vi "Talon Encoder Rotate New.vi"(4 "Right Rotations":dbl, 5 "Right Speed":dbl, 6 "Left Rotations":dbl, 7 "Left Speed":dbl, 9 "RightEncoderMotorRef":T1={"DeviceStatus"={"status"=FALSE, "code"=0, "source"=""}, "Type"=enum."PWM", "PWM"={"PWM Channel"=enum."Invalid", "DeadBand"={"Name"="", "maxPositivePwm"=0, "minPositivePwm"=0, "centerPwm"=0, "maxNegativePwm"=0, "minNegativePwm"=0, "angularRange"=0}}, "CAN"={"Device Number"=0, "Control Mode"=enum."Percent VBus", "Semaphore"=refnum, "Max Vout"=12.0, "TalonSRX Control Mode"=enum."Percent VBus"}, "Invert"=FALSE}, 10 "LeftEncoderMotorRef":T1={"DeviceStatus"={"status"=FALSE, "code"=0, "source"=""}, "Type"=enum."PWM", "PWM"={"PWM Channel"=enum."Invalid", "DeadBand"={"Name"="", "maxPositivePwm"=0, "minPositivePwm"=0, "centerPwm"=0, "maxNegativePwm"=0, "minNegativePwm"=0, "angularRange"=0}}, "CAN"={"Device Number"=0, "Control Mode"=enum."Percent VBus", "Semaphore"=refnum, "Max Vout"=12.0, "TalonSRX Control Mode"=enum."Percent VBus"}, "Invert"=FALSE}, 11 "RobotDriveDevRef":T8={"DevStatus"={"status"=FALSE, "code"=0, "source"=""}, "Motors[]"=[], "Square Inputs"=FALSE, "Max Output"=1.0}) -> (1 "RightEncoderMotorRef":T1={"DeviceStatus"={"status"=FALSE, "code"=0, "source"=""}, "Type"=enum."PWM", "PWM"={"PWM Channel"=enum."Invalid", "DeadBand"={"Name"="", "maxPositivePwm"=0, "minPositivePwm"=0, "centerPwm"=0, "maxNegativePwm"=0, "minNegativePwm"=0, "angularRange"=0}}, "CAN"={"Device Number"=0, "Control Mode"=enum."Percent VBus", "Semaphore"=refnum, "Max Vout"=12.0, "TalonSRX Control Mode"=enum."Percent VBus"}, "Invert"=FALSE}, 2 "LeftEncoderMotorRef":T1={"DeviceStatus"={"status"=FALSE, "code"=0, "source"=""}, "Type"=enum."PWM", "PWM"={"PWM Channel"=enum."Invalid", "DeadBand"={"Name"="", "maxPositivePwm"=0, "minPositivePwm"=0, "centerPwm"=0, "maxNegativePwm"=0, "minNegativePwm"=0, "angularRange"=0}}, "CAN"={"Device Number"=0, "Control Mode"=enum."Percent VBus", "Semaphore"=refnum, "Max Vout"=12.0, "TalonSRX Control Mode"=enum."Percent VBus"}, "Invert"=FALSE}, 3 "RobotDriveDevRef":T8={"DevStatus"={"status"=FALSE, "code"=0, "source"=""}, "Motors[]"=[], "Square Inputs"=FALSE, "Max Output"=1.0})   [LabVIEW 2015]
uses:
  <vilib>/Rock Robotics/WPI/MotorControl/WPI_MotorControlDeviceRef.ctl
  <vilib>/Rock Robotics/WPI/MotorControl/WPI_MotorControlType.ctl
  <vilib>/Rock Robotics/SystemInterfaces/DIO/FPGA_DIOPWMChannel.ctl
  <vilib>/Rock Robotics/WPI/PWM/WPI_PWMDeadband.ctl
  <vilib>/Rock Robotics/WPI/CAN/Jaguar/SubVIs/WPI_CANJaguar_ControlMode.ctl
  <vilib>/Rock Robotics/WPI/CAN/TalonSRX/WPI_CANTalonSRX_APIControlMode.ctl
  <vilib>/Rock Robotics/WPI/RobotDrive/WPI_RobotDriveDevRef.ctl
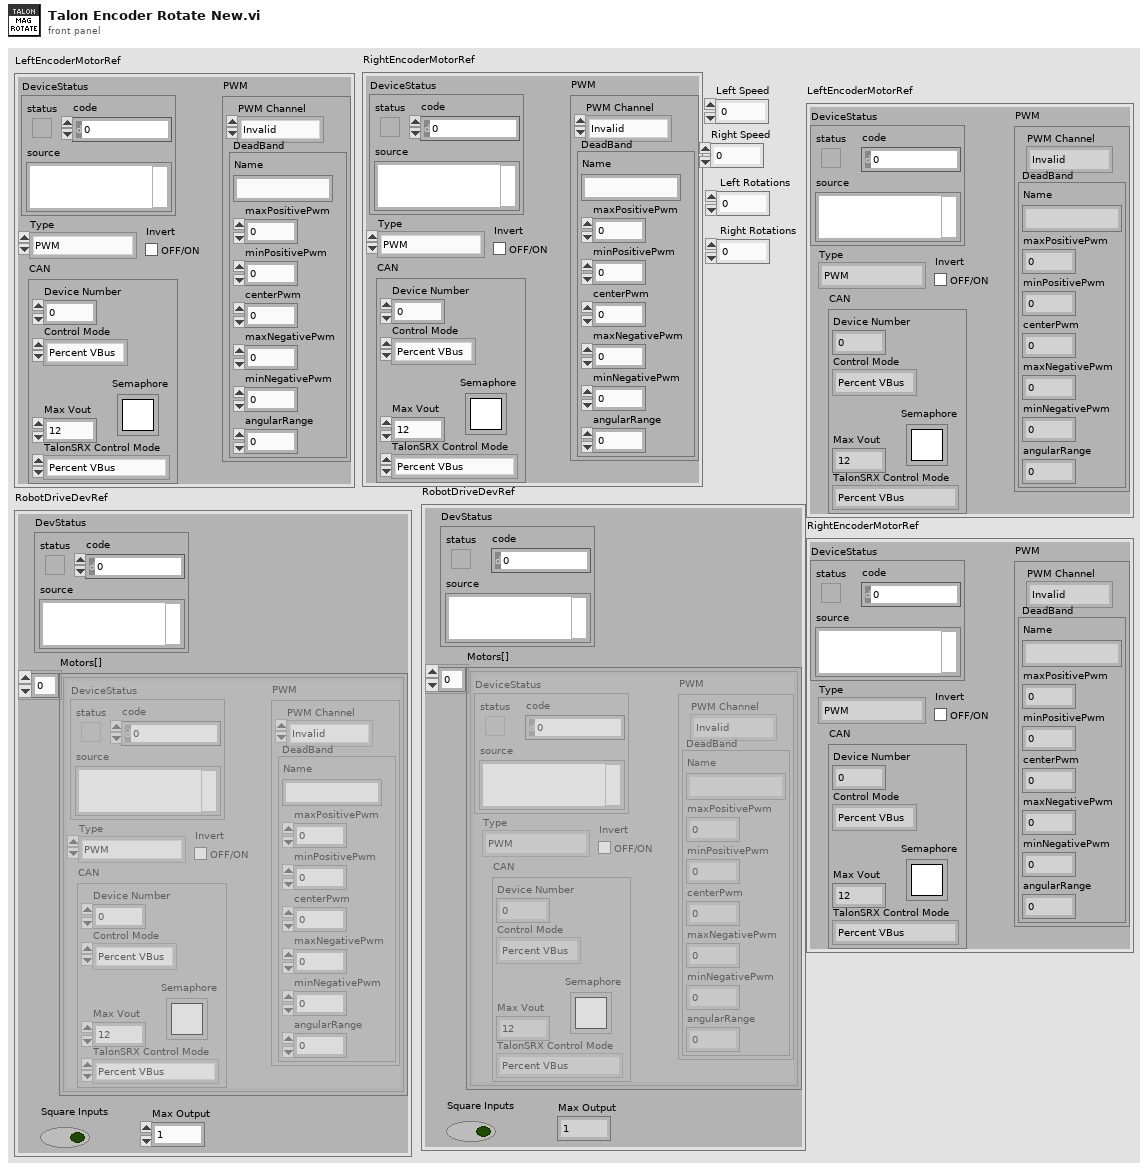
[diagram p1: front panel]
types:
  T1 = typedef "WPI_MotorControlDeviceRef.ctl" = cluster{"DeviceStatus":errorcluster, "Type":T2, "PWM":cluster{"PWM Channel":T3, "DeadBand":T4}, "CAN":cluster{"Device Number":u8, "Control Mode":T5, "Semaphore":T6, "Max Vout":dbl, "TalonSRX Control Mode":T7}, "Invert":bool}
  T2 = typedef "WPI_MotorControlType.ctl" = enum16{"PWM", "CAN", "CANTalonSRX"}
  T3 = typedef "FPGA_DIOPWMChannel.ctl" = enum8{"PWM 0", "PWM 1", "PWM 2", "PWM 3", "PWM 4", "PWM 5", "PWM 6", "PWM 7", "PWM 8", "PWM 9", "PWM MXP 0", "PWM MXP 1", "PWM MXP 2", "PWM MXP 3", "PWM MXP 4", "PWM MXP 5", "PWM MXP 6", "PWM MXP 7", "PWM MXP 8", "PWM MXP 9", "Invalid"}
  T4 = typedef "WPI_PWMDeadband.ctl" = cluster{"Name":string, "maxPositivePwm":i32, "minPositivePwm":i32, "centerPwm":i32, "maxNegativePwm":i32, "minNegativePwm":i32, "angularRange":u16}
  T5 = typedef "WPI_CANJaguar_ControlMode.ctl" = enum8{"Percent VBus", "Current", "Speed", "Position", "Voltage"}
  T6 = typedef "Semaphore RefNum" = refnum<k1>
  T7 = typedef "WPI_CANTalonSRX_APIControlMode.ctl" = enum8{"Percent VBus", "Speed", "Position", "Slave", "Unchanged / Invalid", "Voltage Compensation", "Current", "Motion Profile"}
  T8 = typedef "WPI_RobotDriveDevRef.ctl" = cluster{"DevStatus":errorcluster, "Motors[]":T1[], "Square Inputs":bool, "Max Output":dbl}
  T9 = typedef "WPI_CANTalonSRX_GlobalStatus.ctl" = cluster{"Applied Throttle":dbl, "Module Enabled":bool, "CAN Error":errorcluster, "Closed Loop Error":dbl, "Forward Limit Switch Closed":bool, "Reverse Limit Switch Closed":bool, "Sensor Position":dbl, "Sensor Velocity":dbl, "Current":dbl, "Sticky Fault - Over Temp":bool, "Sticky Fault - Under Voltage":bool, "Sticky Fault - Forward Limit":bool, "Sticky Fault - Reverse Limit":bool, "Sticky Fault - Forward Soft Limit":bool, "Sticky Fault - Reverse Soft Limit":bool, "Brake is Enabled":bool, "Encoder Position":dbl, "Encoder Velocity":dbl, "Encoder Index Count":dbl, "Encoder A Pin State":bool, "Encoder B Pin State":bool, "Encoder Index Pin State":bool, "Analog In":dbl, "Analog In Velocity":dbl, "Temperature (C)":dbl, "Battery Voltage":dbl, "Control 5 Is Supported":bool, "Current Profile Slot Select":dbl, "Pos Div 8":bool, "Vel Div 4":bool, "Pulse Width Position":i32, "Pulse Width Velocity":i32, "Pulse Width Rise To Rise (us)":i32, "Pulse Width Rise To Fall (us)":i32, "Mot Prof Active Is Under Run":bool, "Mot Prof Active Has Under Run":bool, "Mot Prof Active Is Last":bool, "Mot Prof Active Velocity Only":bool, "Mot Prof Active Is Valid":bool, "Mot Prof Buffer Is Full":bool, "Mot Prof Active Profile Slot Select":i32, "Mot Prof NextID":i32, "Mot Prof Count":i32, "Mot Prof Active Velocity":dbl, "Mot Prof Active Position":dbl, "Mot Prof Output Enable":i32}
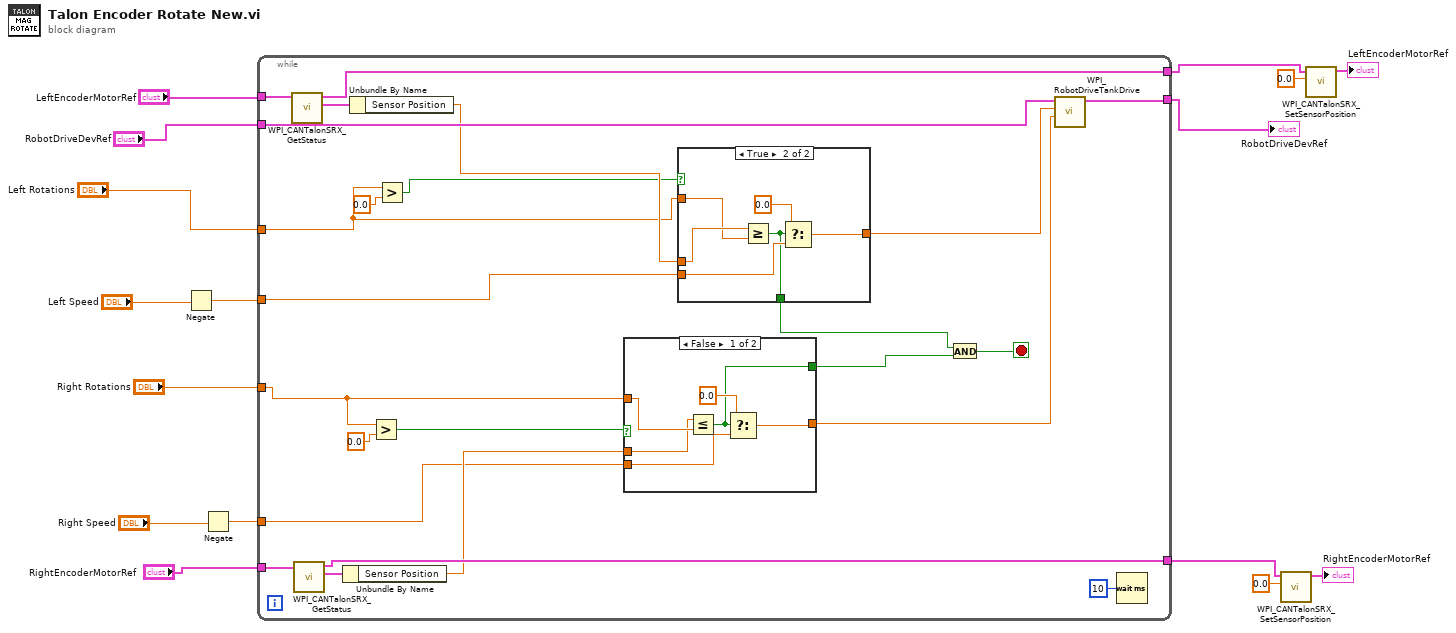
[diagram p0: block diagram]
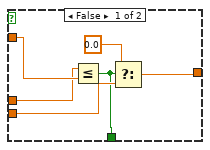
[diagram p2: hidden frame]
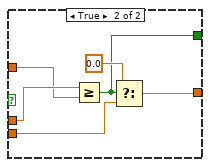
[diagram p3: hidden frame]
diagram:
  n1 = Negate(x="Left Speed") -> (-x=w11:dbl)
  n2 = Negate(x="Right Speed") -> (-x=w1:dbl)
  n3 = while {
    tunnel: [w34] -> w13
    tunnel: "LeftEncoderMotorRef" -> [w36]
    tunnel: "RightEncoderMotorRef" -> [w35]
    tunnel: "RobotDriveDevRef" -> [w33]
    tunnel: "Left Rotations" -> [w19]
    tunnel: w11 -> [w22]
    tunnel: [w32] -> w6
    tunnel: [w31] -> w10
    tunnel: "Right Rotations" -> [w21]
    tunnel: w1 -> [w27]
    stop <- w38 stop-if-true
    n4 = call <vilib>:"WPI_CANTalonSRX_GetStatus.vi"("CAN Talon SRX Ref"=w36) -> ("Talon SRX Status"=w39:T9, "CAN Talon SRX Ref"=w32:T1)  [unwired: 8 in, 1 out]
    n5 = call <vilib>:"WPI_CANTalonSRX_GetStatus.vi"("CAN Talon SRX Ref"=w35) -> ("Talon SRX Status"=w40:T9, "CAN Talon SRX Ref"=w31:T1)  [unwired: 8 in, 1 out]
    n6 = Unbundle By Name(w40) -> ("Sensor Position"=w29:dbl)
    n7 = Unbundle By Name(w39) -> ("Sensor Position"=w24:dbl)
    n8 = Greater?(x=w21, y=0.0) -> (0:w26:bool)
    n9 = Greater?(x=w19, y=0.0) -> (0:w20:bool)
    n10 = case shown="False" w26 {
      tunnel: w21 -> [w57 w63]
      tunnel: w29 -> [w56 w64]
      tunnel: w27 -> [w55 w61]
      tunnel: [w54 w60] -> w25
      tunnel: [w53 w59] -> w17
      frame False {
        n11 = Less Or Equal?(x=w56, y=w57) -> (x <= y?=w53:bool)
        n12 = Select(t=0.0, s=w53, f=w55) -> (s? t:f=w54:dbl)
      }
      frame True {
        n13 = Greater Or Equal?(x=w64, y=w63) -> (x >= y?=w59:bool)
        n14 = Select(t=0.0, s=w59, f=w61) -> (s? t:f=w60:dbl)
      }
    }
    n15 = case shown="True" w20 {
      tunnel: w19 -> [w45 w51]
      tunnel: w24 -> [w44 w52]
      tunnel: w22 -> [w43 w49]
      tunnel: [w42 w48] -> w23
      tunnel: [w41 w47] -> w18
      frame False {
        n16 = Less Or Equal?(x=w44, y=w45) -> (x <= y?=w41:bool)
        n17 = Select(t=0.0, s=w41, f=w43) -> (s? t:f=w42:dbl)
      }
      frame True {
        n18 = Greater Or Equal?(x=w52, y=w51) -> (x >= y?=w47:bool)
        n19 = Select(t=0.0, s=w47, f=w49) -> (s? t:f=w48:dbl)
      }
    }
    n20 = And(x=w18, y=w17) -> (x .and. y?=w38:bool)
    n21 = call <vilib>:"WPI_RobotDriveTankDrive.vi"("Right axis value"=w25, "Left axis value"=w23, "RobotDriveDevRef"=w33) -> ("RobotDriveDevRef"=w34:T8)  [unwired: 6 in, 2 out]
    n22 = Wait (ms)(milliseconds to wait=u32 10) -> ()  [unwired: 1 out]
  }
  "RobotDriveDevRef" <- w13
  n23 = call <vilib>:"WPI_CANTalonSRX_SetSensorPosition.vi"("New Sensor Position"=0.0, "CAN Talon SRX Ref"=w10) -> ("CAN Talon SRX Ref"=→"RightEncoderMotorRef":T1)  [unwired: 8 in, 1 out]
  n24 = call <vilib>:"WPI_CANTalonSRX_SetSensorPosition.vi"("New Sensor Position"=0.0, "CAN Talon SRX Ref"=w6) -> ("CAN Talon SRX Ref"=→"LeftEncoderMotorRef":T1)  [unwired: 8 in, 1 out]
